vi "Comments Handler.vi"(6 "Marker Options":T1={"Color"=16711680, "pen"={"Width"=2, "Style"=enum."Solid"}, "font"={"Font Name"="System Font", "Size"=16, "Strikeout?"=FALSE, "Italic?"=FALSE, "Underline?"=FALSE, "Outline?"=FALSE, "Shadow?"=FALSE, "Bold?"=FALSE, "FontColor"=6618880}, "caption"=""}, 8 "error in":errorcluster, 9 "Action":T3, 10 "Coords":T2, 11 "GrphChrt":refnum<vi>) -> (0 "error out":errorcluster)   [LabVIEW 2019, in "Graph Tools.lvlib"]
uses:
  Graph Tools.lvlib
  [Comment] Actions.ctl
  <vilib>/Utility/miscctls.llb/LVPoint32TypeDef.ctl
  Selection VIs/controls/MarkerOptions.ctl
  [Comment] Config.ctl
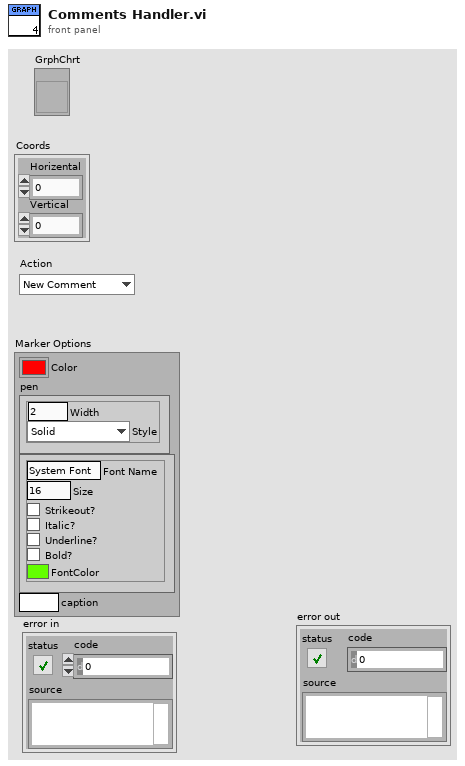
[diagram p1: front panel]
types:
  T1 = typedef "MarkerOptions.ctl" = cluster{"Color":u32, "pen":cluster{"Width":u16, "Style":enum32{"Solid", "Dash", "Dot", "DashDot", "DashDotDot"}}, "font":cluster{"Font Name":string, "Size":i16, "Strikeout?":bool, "Italic?":bool, "Underline?":bool, "Outline?":bool, "Shadow?":bool, "Bold?":bool, "FontColor":u32}, "caption":string}
  T2 = typedef "LVPoint32TypeDef.ctl" = cluster{"Horizental":i32, "Vertical":i32}
  T3 = typedef "Graph Tools.lvlib/[Comment] Actions.ctl" = enum16{"New Comment", "Refresh", "Clear", "Stop", "Test"}
  T4 = typedef "Graph Tools.lvlib/[Comment] Config.ctl" = cluster{"GrphChrt":refnum<vi>, "Position":cluster{"X":dbl, "Y":dbl}, "Comment":string, "Marker Options":T1}
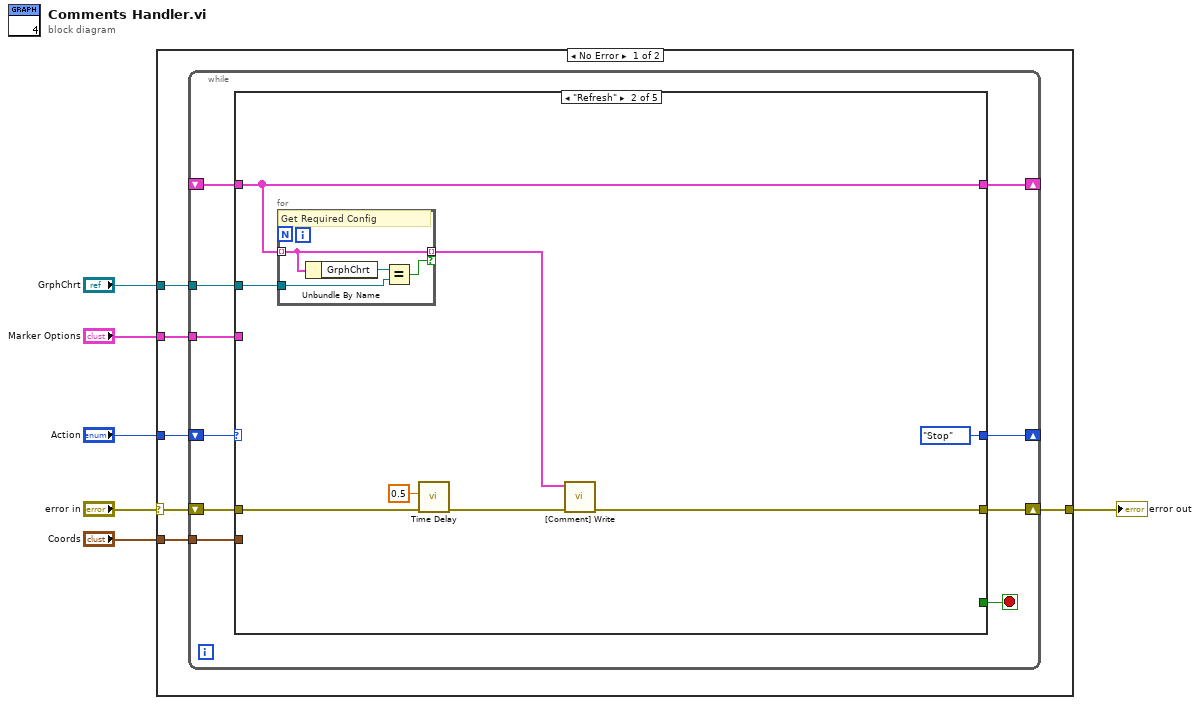
[diagram p0: block diagram]
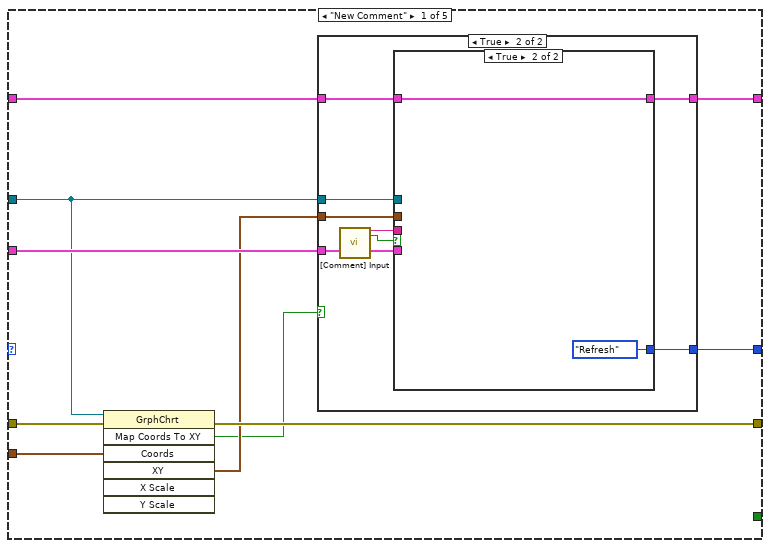
[diagram p2: hidden frame]
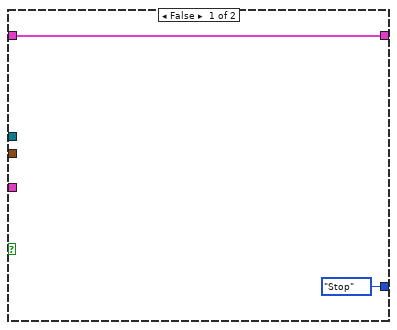
[diagram p3: hidden frame]
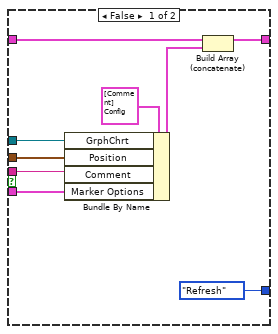
[diagram p4: hidden frame]
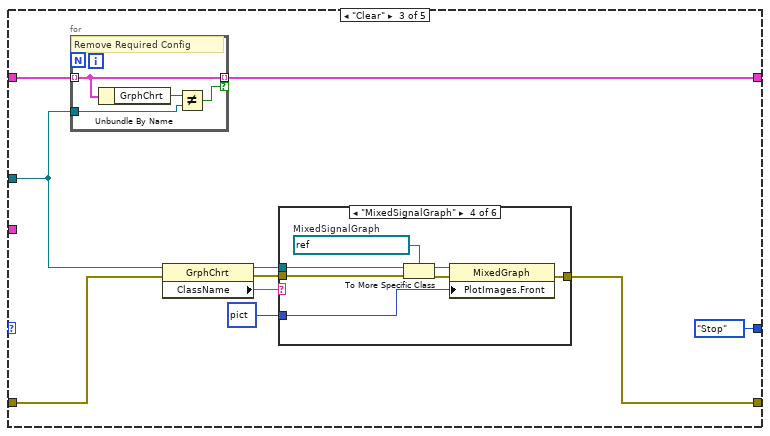
[diagram p5: hidden frame]
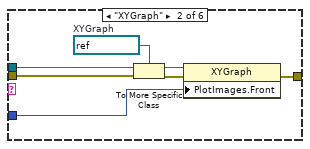
[diagram p7: hidden frame]
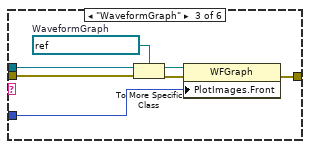
[diagram p8: hidden frame]
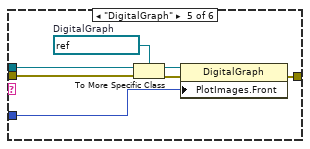
[diagram p9: hidden frame]
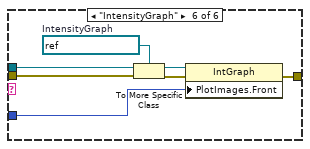
[diagram p10: hidden frame]
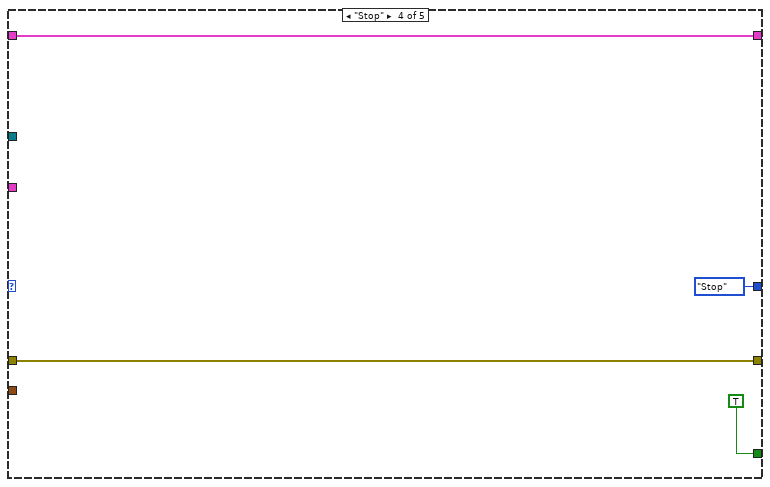
[diagram p11: hidden frame]
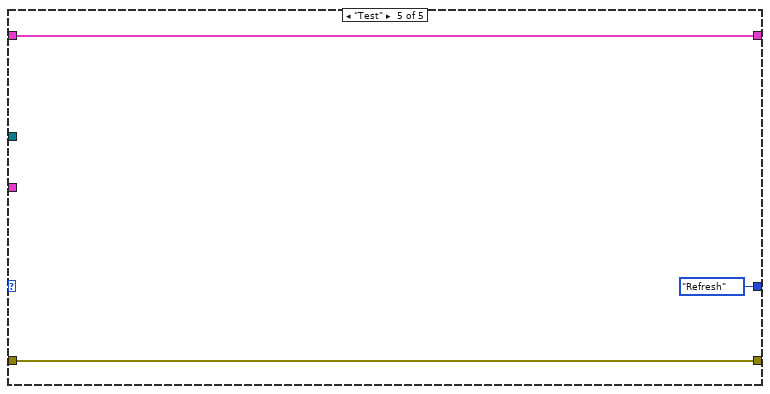
[diagram p12: hidden frame]
diagram:
  n1 = case shown="No Error" "error in" {
    selector: "error in" -> [w11 w123]
    tunnel: "Action" -> [w12 _]
    tunnel: [w10 w123] -> w4
    tunnel: "GrphChrt" -> [w9 _]
    tunnel: "Coords" -> [w8 _]
    tunnel: "Marker Options" -> [w7 _]
    frame No Error {
      n2 = while {
        shift-right: [w21] -> _
        shift-left: _ -> [w20]
        shift-right: [w18] -> w10
        shift-left: w11 -> [w19]
        tunnel: w9 -> [w17]
        tunnel: w8 -> [w16]
        tunnel: w7 -> [w15]
        shift-right: [w14] -> _
        shift-left: w12 -> [w22]
        stop <- w13 stop-if-true
        n3 = case shown="\"Refresh\"" w22 {
          tunnel: [w30 w61 w74 w119 w122] -> w21
          tunnel: w20 -> [w32 w61 w75 w119 w122]
          tunnel: w19 -> [w28 w59 w67 w118 w121]
          tunnel: [w27 w58 w66 w118 w121] -> w18
          tunnel: w17 -> [w24 w56 w68 _ _]
          tunnel: w16 -> [w26 _ _ _ _]
          tunnel: w15 -> [w31 _ _ _ _]
          tunnel: [w29 [Comment]_Actions."Stop" ("Action") [Comment]_Actions."Stop" ("Action") [Comment]_Actions."Stop" ("Action") [Comment]_Actions."Refresh" ("Action")] -> w14
          tunnel: [_ _ _ TRUE _] -> w13
          frame "New Comment" {
            n4 = invoke class="GrphChrt" method="Map Coords To XY"(reference=w24, error in=w28, "Coords"=w26) -> (error out=w27:errorcluster, "Map Coords To XY"=w23:bool, "XY"=w25:cluster{"X":dbl, "Y":dbl})  [unwired: 4 in, 4 out]
            n5 = case shown="True" w23 {
              tunnel: w32 -> [w34 w42]
              tunnel: w31 -> [_ w41]
              tunnel: [w34 w40] -> w30
              tunnel: [[Comment]_Actions."Stop" ("Action") w39] -> w29
              tunnel: w25 -> [_ w36]
              tunnel: w24 -> [_ w35]
              frame False {
              }
              frame True {
                n6 = call "[Comment] Input.vi"() -> ("Comment out"=w38:string, "Canceled?"=w37:bool)  [unwired: 18 in]
                n7 = case shown="True" w37 {
                  tunnel: w42 -> [w51 w52]
                  tunnel: w35 -> [w49 _]
                  tunnel: w36 -> [w48 _]
                  tunnel: w41 -> [w47 _]
                  tunnel: [w46 w52] -> w40
                  tunnel: [[Comment]_Actions."Refresh" ("Action") [Comment]_Actions."Refresh" ("Action")] -> w39
                  tunnel: w38 -> [w43 _]
                  frame False {
                    n8 = Bundle By Name(cluster=T4 {"GrphChrt"=refnum, "Position"={"X"=0.0, "Y"=0.0}, "Comment"="", "Marker Options"={"Color"=16711680, "pen"={"Width"=2, "Style"=enum."Solid"}, "font"={"Font Name"="Arial", "Size"=16, "Strikeout?"=FALSE, "Italic?"=FALSE, "Underline?"=FALSE, "Outline?"=FALSE, "Shadow?"=FALSE, "Bold?"=FALSE, "FontColor"=6618880}, "caption"=""}} ("Graph Comment Config"), "GrphChrt"=w49, "Position"=w48, "Comment"=w43, "Marker Options"=w47) -> (w45:T4)
                    n9 = Build Array (concatenate)(w51, w45) -> (w46:T4[])
                  }
                  frame True {
                  }
                }
              }
            }
          }
          frame "Refresh" {
            n10 = for {
              tunnel: w61 -> [w63] mode=indexing
              tunnel: w56 -> [w64]
              tunnel: [w63] -> w60 mode=indexing if=w62
              # "Get Required Config"
              n11 = Unbundle By Name(w63) -> ("GrphChrt"=w65:refnum<vi>)
              n12 = Equal?(x=w65, y=w64) -> (x = y?=w62:bool)
            }
            n13 = call "Time Delay"("error in (no error)"=w59, "Delay Time (s)"=0.5) -> ("error out"=w55:errorcluster)  [unwired: 9 in]
            n14 = call "[Comment] Write.vi"("error in (no error)"=w55, "Graph Comment Config"=w60) -> ("error out"=w58:errorcluster)  [unwired: 9 in]
          }
          frame "Clear" {
            n15 = for {
              tunnel: w75 -> [w113] mode=indexing
              tunnel: w68 -> [w114]
              tunnel: [w113] -> w74 mode=indexing if=w112
              # "Remove Required Config"
              n16 = Unbundle By Name(w113) -> ("GrphChrt"=w115:refnum<vi>)
              n17 = Not Equal?(x=w115, y=w114) -> (x != y?=w112:bool)
            }
            n18 = property class="GrphChrt"(reference=w68, error in=w67) -> (reference out=w71:refnum<vi>, error out=w70:errorcluster, "ClassName"=w72:string)
            n19 = case shown="\"MixedSignalGraph\"" w72 {
              tunnel: w71 -> [_ w83 w90 w97 w104 w111]
              tunnel: w70 -> [w76 w81 w88 w92 w99 w106]
              tunnel: picture data[5B] ("Picture out") -> [_ w79 w84 w91 w98 w105]
              tunnel: [w76 w77 w86 w94 w101 w108] -> w66
              frame Default {
              }
              frame "XYGraph" {
                w82 = refnum<vi> refnum  # XYGraph
                n20 = To More Specific Class(target class=w82, reference=w83, error in=w81) -> (specific class reference=w80:refnum<vi>, error out=w78:errorcluster)
                n21 = property class="XYGraph"(reference=w80, error in=w78, "PlotImages.Front"=w79) -> (error out=w77:errorcluster)  [unwired: 1 out]
              }
              frame "WaveformGraph" {
                w89 = refnum<vi> refnum  # WaveformGraph
                n22 = To More Specific Class(target class=w89, reference=w90, error in=w88) -> (specific class reference=w87:refnum<vi>, error out=w85:errorcluster)
                n23 = property class="WFGraph"(reference=w87, error in=w85, "PlotImages.Front"=w84) -> (error out=w86:errorcluster)  [unwired: 1 out]
              }
              frame "MixedSignalGraph" {
                w96 = refnum<vi> refnum  # MixedSignalGraph
                n24 = To More Specific Class(target class=w96, reference=w97, error in=w92) -> (specific class reference=w95:refnum<vi>, error out=w93:errorcluster)
                n25 = property class="MixedGraph"(reference=w95, error in=w93, "PlotImages.Front"=w91) -> (error out=w94:errorcluster)  [unwired: 1 out]
              }
              frame "DigitalGraph" {
                w103 = refnum<vi> refnum  # DigitalGraph
                n26 = To More Specific Class(target class=w103, reference=w104, error in=w99) -> (specific class reference=w102:refnum<vi>, error out=w100:errorcluster)
                n27 = property class="DigitalGraph"(reference=w102, error in=w100, "PlotImages.Front"=w98) -> (error out=w101:errorcluster)  [unwired: 1 out]
              }
              frame "IntensityGraph" {
                w110 = refnum<vi> refnum  # IntensityGraph
                n28 = To More Specific Class(target class=w110, reference=w111, error in=w106) -> (specific class reference=w109:refnum<vi>, error out=w107:errorcluster)
                n29 = property class="IntGraph"(reference=w109, error in=w107, "PlotImages.Front"=w105) -> (error out=w108:errorcluster)  [unwired: 1 out]
              }
            }
          }
          frame "Stop" {
          }
          frame "Test" {
          }
        }
      }
    }
    frame Error {
    }
  }
  "error out" <- w4
